vi "SENS_CORR_CCH_ACQ.vi"(0 "VISA IN":refnum<visa-resource-name>, 1 "Ecal":string(combo)="ECAL1", 2 "Char":string, 5 "error in":errorcluster, 7 "Channel":i32=1) -> (14 "VISA Out":refnum<visa-resource-name>, 19 "error out":errorcluster)   [LabVIEW 2018, in "PNA-X.lvlib"]
doc: "SENSe<cnum>:CORRection:CCHeck[:ACQuire] <mod>[,char] \n(Write-only) Reads the 'confidence data' associated with the specified ECal module and puts it into \nmemory. The measurement is selected using SENS:CORR:CCH:PAR. This command is compatible \nwith *OPC. \nParameters \n<cnum> Any existing channel number. If unspecified, value is set to 1. \n<mod> ECAL Module that contains the confidence data. Choose from: \nECAL1 \n..through.. \nECAL8 \n[char] Optional argument. Specifies which characterization within the ECal module \nthat the confidence data will be read from. \nCHAR0 Factory characterization (data that was stored in the ECal module by \n1624\n\nAgilent). Default if not specified. \nCHAR1 User characterization #1 \nCHAR2 User characterization #2 \nCHAR3 User characterization #3 \nCHAR4 User characterization #4 \nCHAR5 User characterization #5 \nExamples SENS:CORR:CCHeck ECAL2 \nsense2:correction:ccheck:acquire ecal1,char1 \nQuery Syntax Not applicable \nDefault Not applicable"
uses:
  PNA-X.lvlib
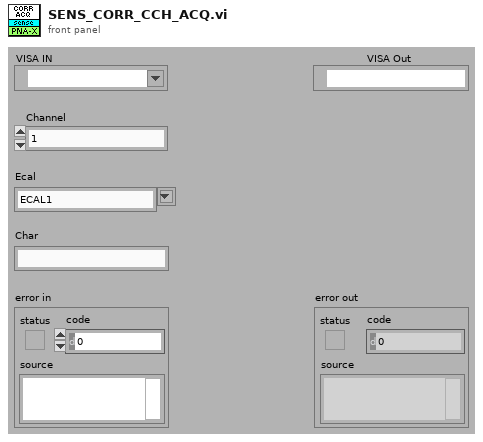
[diagram p1: front panel]
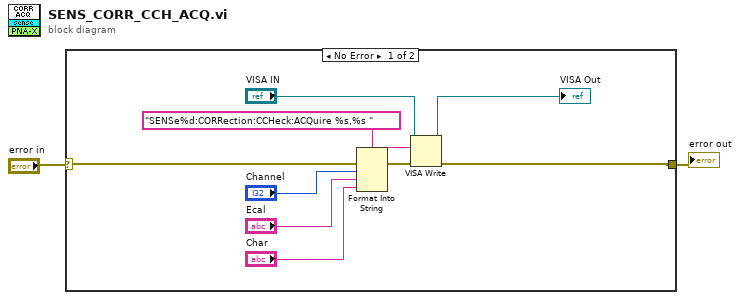
[diagram p0: block diagram]
diagram:
  n1 = case shown="No Error" "error in" {
    selector: "error in" -> [w12 w13]
    tunnel: [w7 w13] -> w1
    frame No Error {
      n2 = Format Into String(format string="SENSe%d:CORRection:CCHeck:ACQuire %s,%s " ("Cmdline"), error in=w12, "Channel", "Ecal", "Char") -> (resulting string=w10:string, error out=w11:errorcluster)  [unwired: 1 in]
      n3 = VISA Write(VISA resource name="VISA IN", write buffer=w10, error in (no error)=w11) -> (VISA resource name out=→"VISA Out":refnum<visa-resource-name>, error out=w7:errorcluster)  [unwired: 1 out]
    }
    frame Error {
    }
  }
  "error out" <- w1
